vi "Draw Menu.vi"(4 "error in (no error)":errorcluster, 5 "Tree Items":T1(array[cluster]), 6 "VI Reference":refnum<vi>, 7 "TreeControl in":refnum<vi>) -> (0 "error out":errorcluster)   [LabVIEW 2015, in "Startup Processes.lvlib"]
uses:
  Startup Processes.lvlib
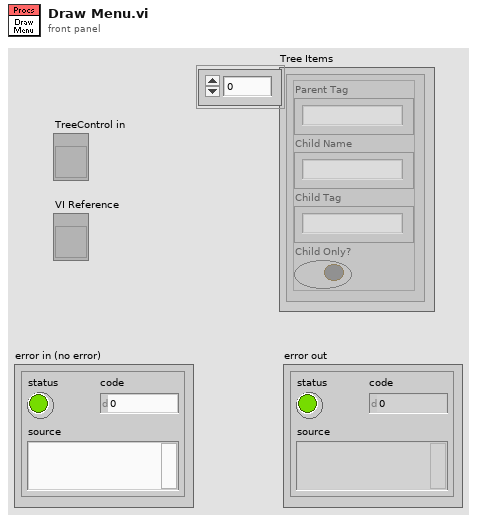
[diagram p1: front panel]
types:
  T1 = cluster{"Parent Tag":string, "Child Name":string, "Child Tag":string, "Child Only?":bool}[]
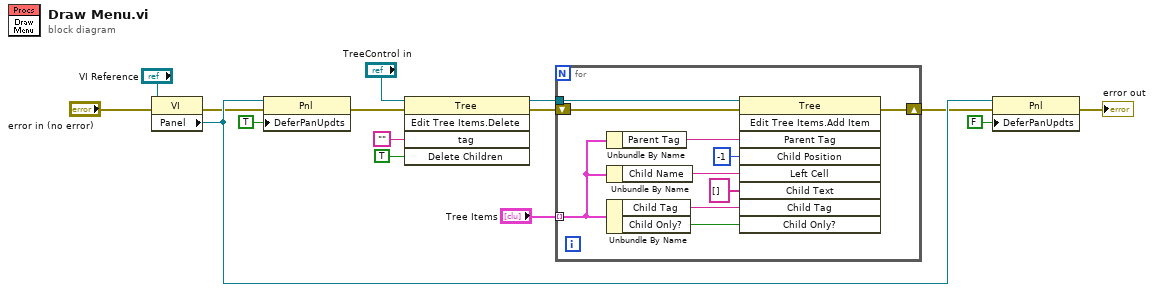
[diagram p0: block diagram]
diagram:
  n1 = property class="VI"(reference="VI Reference", error in="error in (no error)") -> (error out=w11:errorcluster, "Panel"=w15:refnum<vi>)  [unwired: 1 out]
  n2 = property class="Pnl"(reference=w15, error in=w11, "DeferPanUpdts"=TRUE ("Defer Panel Updates")) -> (error out=w3:errorcluster)  [unwired: 1 out]
  n3 = invoke on="Invoke Node" class="Tree" method="Edit Tree Items.Delete"(reference="TreeControl in", error in=w3, "tag"="", "Delete Children"=TRUE) -> (reference out=w2:refnum<vi>, error out=w1:errorcluster)  [unwired: 1 in, 3 out]
  n4 = for {
    tunnel: "Tree Items" -> [w20] mode=indexing
    shift-right: [w24] -> w5
    shift-left: w1 -> [w25]
    tunnel: w2 -> [w16]
    n5 = Unbundle By Name(w20) -> ("Parent Tag"=w23:string)
    n6 = Unbundle By Name(w20) -> ("Child Name"=w21:string)
    n7 = Unbundle By Name(w20) -> ("Child Tag"=w19:string, "Child Only?"=w17:bool)
    n8 = invoke on="Invoke Node" class="Tree" method="Edit Tree Items.Add Item"(reference=w16, error in=w25, "Parent Tag"=w23, "Child Position"=-1, "Left Cell"=w21, "Child Text"=string[] [], "Child Tag"=w19, "Child Only?"=w17) -> (error out=w24:errorcluster)  [unwired: 1 in, 8 out]
  }
  n9 = property class="Pnl"(reference=w15, error in=w5, "DeferPanUpdts"=FALSE ("Defer Panel Updates")) -> (error out=→"error out":errorcluster)  [unwired: 1 out]
